vi "Prompt INPUT.vi"() -> (0 "Max Current (0:User Specified)":u16(ring) items=["User Specified", "0.707 A", "1.0 A", "1.141 A", "1.732 A"], 1 "Heater Resistance (1:25 Ohm)":u16(ring)=1 items=["25 Ohm"=1, "50 Ohm"=2], 2 "Input (0:None)":u16(ring)=1 items=["None", "A", "B"], 3 "Cancelled?":bool)   [LabVIEW 2017]
doc: "Use this template to create a dialog box. This template polls the state of the buttons on the front panel and does not use events. Use the Dialog Using Events template (not available in Base package) to create a dialog box with event handling."
panel:
  in  "Heater Resistance (1:25 Ohm)":u16(ring)=2 items=["25 Ohm"=1, "50 Ohm"=2]
  in  "Max Current (0:User Specified)":u16(ring)=2 items=["User Specified", "0.707 A", "1.0 A", "1.141 A", "1.732 A"]
  in  "Input (0:None)":u16(ring)=1 items=["None", "A", "B"]
  in  "Cancel":bool
  in  "OK":bool
  # "CONFIGURACION DEL LAZO DE CONTROL"
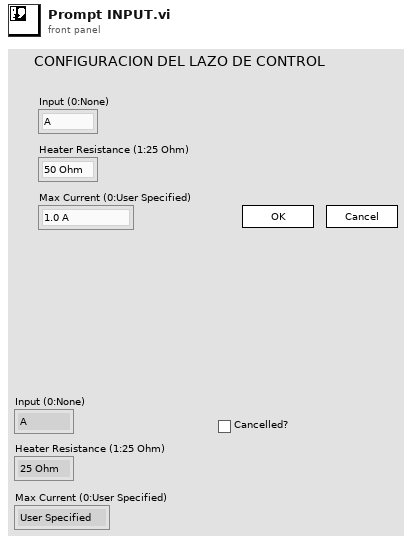
[diagram p1: front panel]
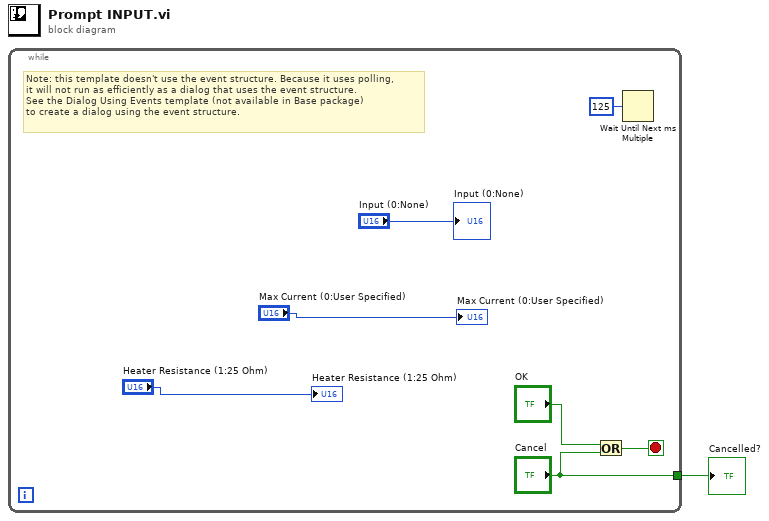
[diagram p0: block diagram]
diagram:
  n1 = while {
    tunnel: ["Cancel"] -> w1
    stop <- w7 stop-if-true
    # "Note: this template doesn't use the event structure. Because it uses polling, \nit will not run as efficiently as a dialog that uses the event structure.\nSee the Dialog Using Events template (not available in Base package) \nto create a dialog using the event structure."
    n2 = Or(x="OK", y="Cancel") -> (x .or. y?=w7:bool)
    n3 = Wait Until Next ms Multiple(millisecond multiple=u32 125) -> ()  [unwired: 1 out]
    "Input (0:None)" <- "Input (0:None)"
    "Max Current (0:User Specified)" <- "Max Current (0:User Specified)"
    "Heater Resistance (1:25 Ohm)" <- "Heater Resistance (1:25 Ohm)"
  }
  "Cancelled?" <- w1
